vi "start.vi"(8 "error in (no error)":errorcluster, 11 "DL090211FrameImageAssembler in":refnum<class "ImageAssemblerDL090211Frame.lvclass">) -> (0 "error out":errorcluster, 3 "DL090211FrameImageAssembler out":refnum<class "ImageAssemblerDL090211Frame.lvclass">)   [LabVIEW 2010, in "ImageAssemblerDL090211Frame.lvclass"]
uses:
  ImageAssemblerDL090211Frame.lvclass
  ImageAssemblerDL090211Scaffold/ImageAssemblerDL090211Scaffold/ImageAssemblerDL090211Scaffold.lvclass
  ImageAssemblerDL090211Frame.lvclass/ImageAssemblerDL090211Frame.ctl
  common/arrays/pixel_raw_data_array.ctl
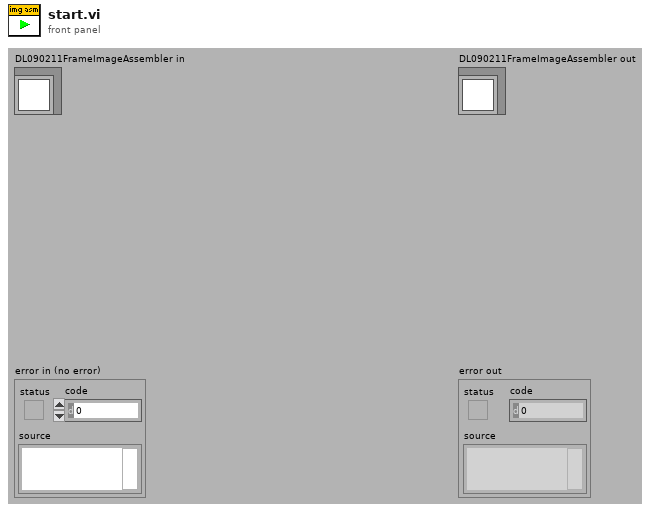
[diagram p1: front panel]
types:
  T1 = typedef "pixel_raw_data_array.ctl" = dbl[][]
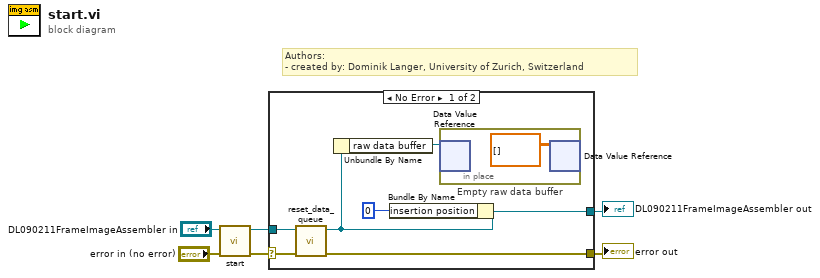
[diagram p0: block diagram]
diagram:
  # "Authors: \n- created by: Dominik Langer, University of Zurich, Switzerland"
  n1 = call-parent "start.vi"("error in (no error)"="error in (no error)", "DL090211ImageAssemblerScaffold in"="DL090211FrameImageAssembler in") -> ("error out"=w1:errorcluster, "DL090211ImageAssemblerScaffold out"=w2:refnum<class "ImageAssemblerDL090211Frame.lvclass">)  [unwired: 8 out]
  n2 = case shown="No Error" w1 {
    selector: w1 -> [w11 w16]
    tunnel: [w10 w16] -> w6
    tunnel: [w13 w15] -> w5
    tunnel: w2 -> [w9 w15]
    frame No Error {
      n3 = call-dynamic "reset_data_queue.vi"("error in (no error)"=w11, "GenericToplevelComponent in"=w9) -> ("error out"=w10:errorcluster, "GenericToplevelComponent out"=w8:refnum<class "ImageAssemblerDL090211Frame.lvclass">)  [unwired: 8 in]
      n4 = Unbundle By Name(w8) -> ("raw data buffer"=w7:refnum<data-value>)
      n5 = Bundle By Name(cluster=w8, "insertion position"=u64 0 ("current insertion coordinate.y")) -> (w13:refnum<class "ImageAssemblerDL090211Frame.lvclass">)
      n6 = in-place "Empty raw data buffer" {
        n7 = in-place-dvr #1(w7) -> ()  [unwired: 2 out]
        n8 = in-place-dvr #1(T1 [] ("data value")) -> ()  [unwired: 2 out]
      }
    }
    frame Error {
    }
  }
  "error out" <- w6
  "DL090211FrameImageAssembler out" <- w5
